vi "solar_cfg Read (Var).vi"(0 "Config Refnum":refnum<data-value>, 1 "Section":string, 2 "Comments (Key,Comment)":cluster{"Key":string, "Comment":string}[](array[cluster]), 5 "Key (\"\")":string, 7 "Variant in":variant, 9 "Include Variant Name? (F)":bool, 11 "error in (no error)":errorcluster, 12 "ArrayDelimiters (1D,2D)":string[](array[string]), 13 "Write If Not Found? (T)":bool=TRUE) -> (4 "dup Config Refnum":refnum<data-value>, 6 "Variant out":variant, 10 "Found?":bool, 15 "error out":errorcluster)   [LabVIEW 2018]
doc: "Reads the values associated with a variant from a specified section in a configuration file. If the Key is empty the variant label is used instead. Set a Comment (#...) to add a description after the key's value. Clusters use the element lables are their key names. Set Enum as Strings to True to use the string item of an enum.\n\nSupported Data Types: \nI8..EXT, Enum, Boolean, String, Path, VISA Reference, Timestamp\n1D & 2D Arrays and Clusters of the data types above.\n\n[Section]\nKey = \"Value\" #Comment"
uses:
  <vilib>/Utility/Data Type/NI_Data Type.lvlib
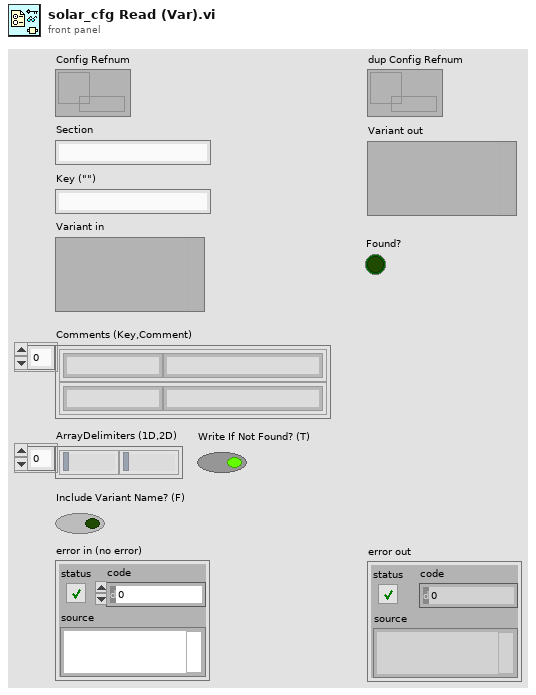
[diagram p1: front panel]
types:
  T1 = typedef "NI_Data Type.lvlib/Data Type.ctl" = enum8{"Invalid Type", "Void", "I8", "I16", "I32", "I64", "U8", "U16", "U32", "U64", "Single Float", "Double Float", "Extended Float", "Single Complex", "Double Complex", "Extended Complex", "Enum U8", "Enum U16", "Enum U32", "Enum U64", "Single Float With Unit", "Double Float With Unit", "Extended Float With Unit", "Single Complex with Unit", "Double Complex with Unit", "Extended Complex with Unit", "Boolean", "String", "Path", "Picture", "Tag", "Array", "Cluster", "Variant", "LV Variant", "Waveform", "Timestamp", "Digital Waveform", "Digital Data", "ExpressData", "Refnum", "External Data", "VI", "Poly VI", "LabVIEW Class Instance", "Fixed Point", "Set Collection", "Map Collection"}
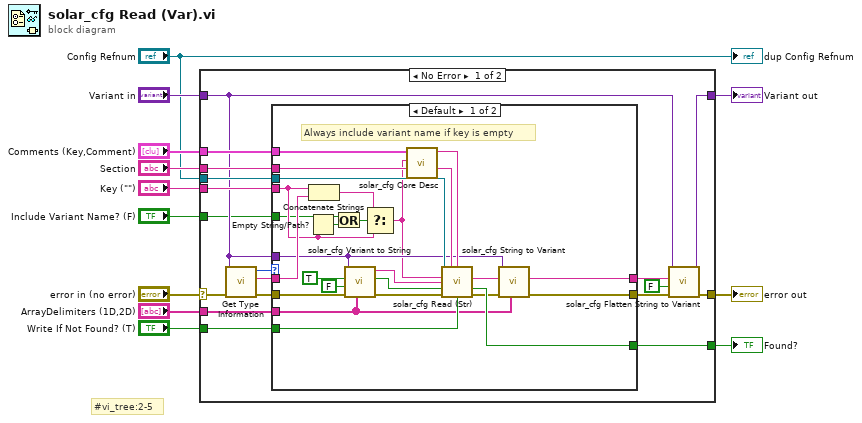
[diagram p0: block diagram]
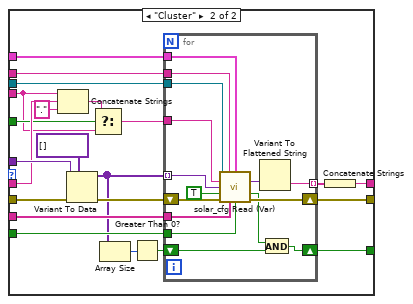
[diagram p2: hidden frame]
diagram:
  # "#vi_tree:2-5"
  n1 = case shown="No Error" "error in (no error)" {
    selector: "error in (no error)" -> [w23 w94]
    tunnel: [w15 w94] -> w10
    tunnel: "Variant in" -> [w18 w93]
    tunnel: [w14 w93] -> w6
    tunnel: "Config Refnum" -> [w28 _]
    tunnel: "Comments (Key,Comment)" -> [w30 _]
    tunnel: "Section" -> [w29 _]
    tunnel: "Key (\"\")" -> [w24 _]
    tunnel: "ArrayDelimiters (1D,2D)" -> [w25 _]
    tunnel: [w27 _] -> w8
    tunnel: "Write If Not Found? (T)" -> [w26 _]
    tunnel: "Include Variant Name? (F)" -> [w13 _]
    frame No Error {
      n2 = call <vilib>:"Get Type Information.vi"("error in (no error)"=w23, "variant"=w18) -> ("error out"=w22:errorcluster, "name"=w20:string, "type"=w21:T1)  [unwired: 5 in, 2 out]
      n3 = case shown="Default" w21 {
        tunnel: w30 -> [w55 w70]
        tunnel: w29 -> [w54 w69]
        tunnel: w28 -> [w53 w74]
        tunnel: [w49 w56] -> w27
        tunnel: w26 -> [w52 w65]
        tunnel: w25 -> [w38 w66]
        tunnel: w24 -> [w34 w61]
        tunnel: w22 -> [w48 w77]
        tunnel: [w39 w60] -> w17
        tunnel: [w40 w76] -> w19
        tunnel: w18 -> [w41 w72]
        tunnel: w20 -> [w50 w67]
        tunnel: w13 -> [w32 w62]
        frame Default {
          # "Always include variant name if key is empty"
          n4 = Empty String/Path?(string/path=w34) -> (empty?=w33:bool)
          n5 = Concatenate Strings(w34, w50) -> (w36:string)
          n6 = Or(x=w32, y=w33) -> (x .or. y?=w31:bool)
          n7 = call "solar_cfg Variant to String.vi"("ArrayDelimiters (1D,2D)"=w38, "error in (no error)"=w48, "Boolean as 0,1? (F)"=FALSE, "Use Enum Names? (F)"=TRUE, "Variant"=w41) -> ("error out"=w43:errorcluster, "Quotes Recommended?"=w44:bool, "String"=w45:string)  [unwired: 3 in, 1 out]
          n8 = Select(t=w36, s=w31, f=w34) -> (s? t:f=w35:string)
          n9 = call "solar_cfg Core Desc.vi"("Key"=w35, "Comments (Key,Comment)"=w55) -> ("Comment"=w51:string)  [unwired: 9 in]
          n10 = call "solar_cfg Read (Str).vi"("Config Refnum"=w53, "Section"=w54, "Comment"=w51, "Key"=w35, "Value in"=w45, "Add Quotes? (T)"=w44, "error in (no error)"=w43, "Write If Not Found? (T)"=w52) -> ("Value out (quotes removed)"=w37:string, "Found?"=w49:bool, "error out"=w42:errorcluster)  [unwired: 4 in, 1 out]
          n11 = call "solar_cfg String to Variant.vi"("ArrayDelimiters (1D,2D)"=w38, "error in (no error)"=w42, "String"=w37, "Variant in"=w41) -> ("error out"=w40:errorcluster, "Variant (Binary)"=w39:string)  [unwired: 5 in, 1 out]
        }
        frame "Cluster" {
          n12 = Concatenate Strings(w61, w67, "." ("string")) -> (w64:string)
          n13 = Variant To Data(error in=w77, type=variant[] [], Variant=w72) -> (data=w59:variant[], error out=w73:errorcluster)
          n14 = Select(t=w64, s=w62, f=w61) -> (s? t:f=w63:string)
          n15 = Array Size(array=w59) -> (size(s)=w58:i32)
          n16 = Greater Than 0?(x=w58) -> (x > 0?=w57:bool)
          n17 = for {
            tunnel: [w90] -> w75 mode=indexing
            tunnel: w74 -> [w89]
            shift-right: [w92] -> w76
            shift-left: w73 -> [w88]
            tunnel: w70 -> [w86]
            tunnel: w69 -> [w87]
            tunnel: w63 -> [w85]
            tunnel: w59 -> [w84] mode=indexing
            tunnel: w66 -> [w83]
            tunnel: w65 -> [w82]
            shift-right: [w80] -> w56
            shift-left: w57 -> [w79]
            n18 = call "solar_cfg Read (Var).vi"("Config Refnum"=w89, "Section"=w87, "Comments (Key,Comment)"=w86, "Key (\"\")"=w85, "Variant in"=w84, "Include Variant Name? (F)"=TRUE ("Include Prefix? (T)"), "error in (no error)"=w88, "ArrayDelimiters (1D,2D)"=w83, "Write If Not Found? (T)"=w82) -> ("Variant out"=w91:variant, "Found?"=w81:bool, "error out"=w92:errorcluster)  [unwired: 3 in, 1 out]
            n19 = Variant To Flattened String(Variant=w91) -> (data string=w90:string)  [unwired: 1 out]
            n20 = And(x=w81, y=w79) -> (x .and. y?=w80:bool)
          }
          n21 = Concatenate Strings(w75) -> (w60:string)
        }
      }
      n22 = call "solar_cfg Flatten String to Variant.vi"("error in (no error)"=w19, "Keep Attributes? (F)"=FALSE, "Data String"=w17, "Variant in"=w18) -> ("error out"=w15:errorcluster, "Variant out"=w14:variant)  [unwired: 5 in, 1 out]
    }
    frame Error {
    }
  }
  "error out" <- w10
  "Variant out" <- w6
  "Found?" <- w8
  "dup Config Refnum" <- "Config Refnum"
